vi "WordValue2WordStr.vi"(8 "error in":errorcluster, 11 "WordValue":i32) -> (0 "error out":errorcluster, 3 "WordStr":string)   [LabVIEW 2016, in "Motor Base.lvlib" / "Motor Base.lvclass"]
uses:
  Motor Base.lvclass
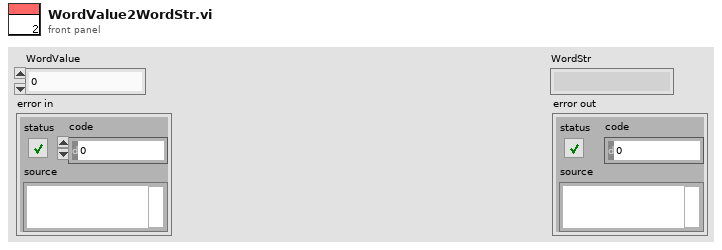
[diagram p1: front panel]
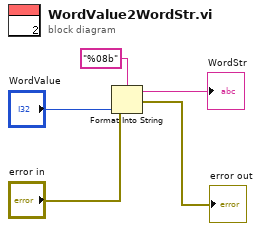
[diagram p0: block diagram]
diagram:
  n1 = Format Into String(format string="%08b", error in="error in", "WordValue") -> (resulting string=→"WordStr":string, error out=→"error out":errorcluster)  [unwired: 1 in]
